vi "Send Template.vi"(5 "Message Type":refnum<class "Abstract Message Template.lvclass">, 7 "Message Priority (Normal)":T1=enum."Normal", 8 "error in (no error)":errorcluster, 11 "Message Enqueuer":refnum<class "Message Enqueuer.lvclass">) -> (0 "error out":errorcluster, 3 "Message Enqueuer out":refnum<class "Message Enqueuer.lvclass">)   [LabVIEW 2020, in "Abstract Message Template.lvclass"]
doc: "This VI sends the message to an actor."
uses:
  Abstract Message Template.lvclass
  Abstract Message Template.lvclass/Abstract Message Template.ctl
  vi.lib/ActorFramework/Message/Message.lvclass
  vi.lib/ActorFramework/Message Enqueuer/Message Enqueuer.lvclass
  vi.lib/ActorFramework/Message Enqueuer/Message Priority.ctl
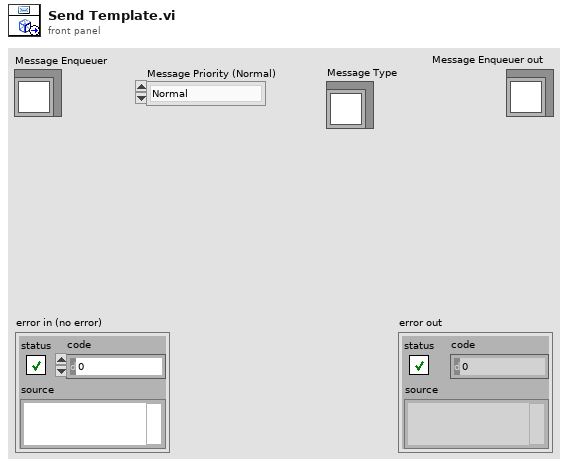
[diagram p1: front panel]
types:
  T1 = typedef "Actor Framework.lvlib/Message Enqueuer.lvclass/Message Priority.ctl" = enum16{"Low", "Normal", "High"}
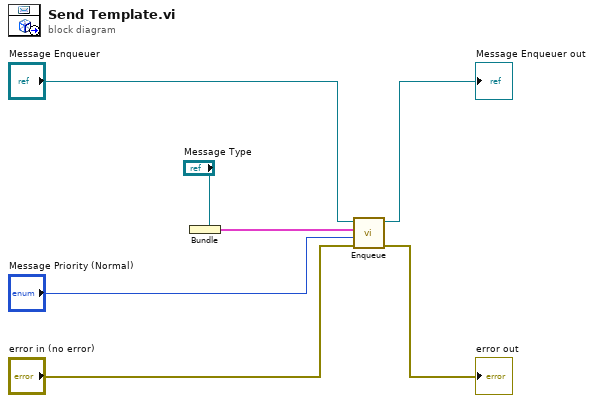
[diagram p0: block diagram]
diagram:
  n1 = Bundle(cluster="Message Type") -> (w3:cluster{void})  [unwired: 1 in]
  n2 = call "Enqueue.vi"("error in (no error)"="error in (no error)", "Message Priority (Normal)"="Message Priority (Normal)", "Message"=w3, "Message Enqueuer in"="Message Enqueuer") -> ("error out"=→"error out":errorcluster, "Message Enqueuer out"=→"Message Enqueuer out":refnum<class "Message Enqueuer.lvclass">)  [unwired: 6 in]
